vi "HEWH Flow Adjust Draw States.vi"(4 "GPM Target":T3=3.0 format="%.2f", 5 "Loop Rate":dbl, 6 "Elapsed Time (Sec)":dbl, 7 "Flow Selector":T1, 8 "Error In":errorcluster, 9 "Gallon Target":T3 format="%.2f", 10 "Core HEWH Data in":T4={"Scan Rate Adjust"=0.0, "Draw Count"=0, "Test Patten Setup"={"Total Gallons Schedule"=[], "PRAT/RLT Sequence"=[{"Sequence #"=1.0, "Cycles"=35, "Mode Setting"="", "Flow Rate (GPM)"=0.0, "Temperature (F)"=0.0, "Reset Timer"=FALSE, "Use Temp Decline Method"=FALSE, "Terminate Condition"=enum."C1-Terminate Draw @ Gallon Mark", "Condition Value #1"=0.0, "UE"=FALSE, "LE"=FALSE, "Comp"=FALSE, "Fan"=FALSE, "Test End Time (Sec)"=0.0, "Purge Until Cutout"=FALSE, "Start Conditions"=enum."Heat Source Cutout", "Condition Value #2"=0.0, "Remove Power"=FALSE, "Time"=0.0, "Check Special Cond."=enum."SC1-Do Nothing", "Condition#"=enum."C1", "Draw Flags"=enum."N/A", "Data Processing Delay (FHD 15sec, UEF 5 Sec)"=0.0, "Test Complete"=FALSE, "User Setpoint"=0.0, "Tank Setpoint"=0.0}, {"Sequence #"=2.0, "Cycles"=15, "Mode Setting"="", "Flow Rate (GPM)"=0.0, "Temperature (F)"=0.0, "Reset Timer"=FALSE, "Use Temp Decline Method"=FALSE, "Terminate Condition"=enum."C1-Terminate Draw @ Gallon Mark", "Condition Value #1"=0.0, "UE"=FALSE, "LE"=FALSE, "Comp"=FALSE, "Fan"=FALSE, "Test End Time (Sec)"=0.0, "Purge Until Cutout"=FALSE, "Start Conditions"=enum."Heat Source Cutout", "Condition Value #2"=0.0, "Remove Power"=FALSE, "Time"=0.0, "Check Special Cond."=enum."SC1-Do Nothing", "Condition#"=enum."C1", "Draw Flags"=enum."N/A", "Data Processing Delay (FHD 15sec, UEF 5 Sec)"=0.0, "Test Complete"=FALSE, "User Setpoint"=0.0, "Tank Setpoint"=0.0}, {"Sequence #"=3.0, "Cycles"=35, "Mode Setting"="", "Flow Rate (GPM)"=0.0, "Temperature (F)"=0.0, "Reset Timer"=FALSE, "Use Temp Decline Method"=FALSE, "Terminate Condition"=enum."C1-Terminate Draw @ Gallon Mark", "Condition Value #1"=0.0, "UE"=FALSE, "LE"=FALSE, "Comp"=FALSE, "Fan"=FALSE, "Test End Time (Sec)"=0.0, "Purge Until Cutout"=FALSE, "Start Conditions"=enum."Heat Source Cutout", "Condition Value #2"=0.0, "Remove Power"=FALSE, "Time"=0.0, "Check Special Cond."=enum."SC1-Do Nothing", "Condition#"=enum."C1", "Draw Flags"=enum."N/A", "Data Processing Delay (FHD 15sec, UEF 5 Sec)"=0.0, "Test Complete"=FALSE, "User Setpoint"=0.0, "Tank Setpoint"=0.0}, {"Sequence #"=4.0, "Cycles"=15, "Mode Setting"="", "Flow Rate (GPM)"=0.0, "Temperature (F)"=0.0, "Reset Timer"=FALSE, "Use Temp Decline Method"=FALSE, "Terminate Condition"=enum."C1-Terminate Draw @ Gallon Mark", "Condition Value #1"=0.0, "UE"=FALSE, "LE"=FALSE, "Comp"=FALSE, "Fan"=FALSE, "Test End Time (Sec)"=0.0, "Purge Until Cutout"=FALSE, "Start Conditions"=enum."Heat Source Cutout", "Condition Value #2"=0.0, "Remove Power"=FALSE, "Time"=0.0, "Check Special Cond."=enum."SC1-Do Nothing", "Condition#"=enum."C1", "Draw Flags"=enum."N/A", "Data Processing Delay (FHD 15sec, UEF 5 Sec)"=0.0, "Test Complete"=FALSE, "User Setpoint"=0.0, "Tank Setpoint"=0.0}, {"Sequence #"=5.0, "Cycles"=35, "Mode Setting"="", "Flow Rate (GPM)"=0.0, "Temperature (F)"=0.0, "Reset Timer"=FALSE, "Use Temp Decline Method"=FALSE, "Terminate Condition"=enum."C1-Terminate Draw @ Gallon Mark", "Condition Value #1"=0.0, "UE"=FALSE, "LE"=FALSE, "Comp"=FALSE, "Fan"=FALSE, "Test End Time (Sec)"=0.0, "Purge Until Cutout"=FALSE, "Start Conditions"=enum."Heat Source Cutout", "Condition Value #2"=0.0, "Remove Power"=FALSE, "Time"=0.0, "Check Special Cond."=enum."SC1-Do Nothing", "Condition#"=enum."C1", "Draw Flags"=enum."N/A", "Data Processing Delay (FHD 15sec, UEF 5 Sec)"=0.0, "Test Complete"=FALSE, "User Setpoint"=0.0, "Tank Setpoint"=0.0}, {"Sequence #"=6.0, "Cycles"=15, "Mode Setting"="", "Flow Rate (GPM)"=0.0, "Temperature (F)"=0.0, "Reset Timer"=FALSE, "Use Temp Decline Method"=FALSE, "Terminate Condition"=enum."C1-Terminate Draw @ Gallon Mark", "Condition Value #1"=0.0, "UE"=FALSE, "LE"=FALSE, "Comp"=FALSE, "Fan"=FALSE, "Test End Time (Sec)"=0.0, "Purge Until Cutout"=FALSE, "Start Conditions"=enum."Heat Source Cutout", "Condition Value #2"=0.0, "Remove Power"=FALSE, "Time"=0.0, "Check Special Cond."=enum."SC1-Do Nothing", "Condition#"=enum."C1", "Draw Flags"=enum."N/A", "Data Processing Delay (FHD 15sec, UEF 5 Sec)"=0.0, "Test Complete"=FALSE, "User Setpoint"=0.0, "Tank Setpoint"=0.0}, {"Sequence #"=7.0, "Cycles"=35, "Mode Setting"="", "Flow Rate (GPM)"=0.0, "Temperature (F)"=0.0, "Reset Timer"=FALSE, "Use Temp Decline Method"=FALSE, "Terminate Condition"=enum."C1-Terminate Draw @ Gallon Mark", "Condition Value #1"=0.0, "UE"=FALSE, "LE"=FALSE, "Comp"=FALSE, "Fan"=FALSE, "Test End Time (Sec)"=0.0, "Purge Until Cutout"=FALSE, "Start Conditions"=enum."Heat Source Cutout", "Condition Value #2"=0.0, "Remove Power"=FALSE, "Time"=0.0, "Check Special Cond."=enum."SC1-Do Nothing", "Condition#"=enum."C1", "Draw Flags"=enum."N/A", "Data Processing Delay (FHD 15sec, UEF 5 Sec)"=0.0, "Test Complete"=FALSE, "User Setpoint"=0.0, "Tank Setpoint"=0.0}, {"Sequence #"=8.0, "Cycles"=15, "Mode Setting"="", "Flow Rate (GPM)"=0.0, "Temperature (F)"=0.0, "Reset Timer"=FALSE, "Use Temp Decline Method"=FALSE, "Terminate Condition"=enum."C1-Terminate Draw @ Gallon Mark", "Condition Value #1"=0.0, "UE"=FALSE, "LE"=FALSE, "Comp"=FALSE, "Fan"=FALSE, "Test End Time (Sec)"=0.0, "Purge Until Cutout"=FALSE, "Start Conditions"=enum."Heat Source Cutout", "Condition Value #2"=0.0, "Remove Power"=FALSE, "Time"=0.0, "Check Special Cond."=enum."SC1-Do Nothing", "Condition#"=enum."C1", "Draw Flags"=enum."N/A", "Data Processing Delay (FHD 15sec, UEF 5 Sec)"=0.0, "Test Complete"=FALSE, "User Setpoint"=0.0, "Tank Setpoint"=0.0}], "Current Sequence Index"=0}, "HEWH Specific DAQ"={"HEWH Data"={"HEWH Standard"={"Voltage (Volts)"=0.0, "Current (Amps)"=0.0, "Power (Watts)"=0.0, "WattHours (Wh)"=0.0, "TC Tree (AVG)"=0.0, "Flow Rate (GPM)"=0.0, "Gallons (Gal)"=0.0, "RTD Out (Deg F)"=0.0, "RTD In (Deg F)"=0.0, "RTD Amb (Deg F)"=0.0, "TC Down"=0.0, "UE Event Lead"=0, "LE Event Lead"=0, "TC Tree Array"=[]}, "PRAT"={"Power (Watts) A"=4192.0, "Power (Watts) B"=4192.0, "Power (Watts) C"=4192.0, "Power (Watts) D"=4192.0, "TC1"=0.0, "TC2"=0.0, "TC3"=0.0, "TC4"=0.0, "WattHours (Wh) A"=4192.0, "WattHours (Wh) B"=4192.0, "WattHours (Wh) C"=4192.0, "WattHours (Wh) D"=4192.0, "Ambient"=0.0, "Extra Temp"=0.0}, "Additional Power Data"={"Vthd"=236.2, "Frequency (Hz)"=236.2, "Apparent Power (VA)"=236.2, "Power Factor"=236.2, "Current Crest Factor"=236.2, "Voltage Crest Factor"=236.2, "Integration Time (sec)"=236.2}}, "Flow Valve % Open"=0.0, "Power State"={"UE"=FALSE, "LE"=FALSE, "COMP"=FALSE, "FANS"=FALSE}, "Power Analyzer"=enum."", "Flow Valve uA Output"=0, "Gallons Start (Gal)"=0.0}, "Test Output Data"={"PreDraw Data Table"=[], "Data Table"=[], "MW100 TC Headers"=[]}, "Calc and Calibration"={"Mean SD Var Max Min Array"=[], "Draw Statistics (DBL)"=[], "Calibration Coefficients DBL"=[], "Start Gallons"=0.0, "Starting Temp Decline"=0.0, "K-Factor (Temperature)"=0.0, "All Draw Stats"=[], "RTD Terminate Value"=0.0, "K-Factor (Flow)"=0.0, "Intellifaucet Type"="", "Thermal Stabil Array"=[], "Gas Thermal Stabil Complete"=FALSE, "Therm Reset Cmpt 1"=FALSE, "Therm Reset Cmpt 2"=FALSE, "Last Flow Rate (Therm)"=0.0, "State"=enum."State 1", "Gas Thermal Time"=0.0, "Target Rate (Thermal)"=0.0, "Thermal - Final"=[], "State5 Gal Water"=0.0, "State 5 Gal Gas"=0.0, "Intellif Open < 1"=0.0, "Intellif Open < 1.7"=0.0, "Intellif Open < 2.2"=0.0, "Intellif Open > 2.2"=0.0, "End of Draw\nComparison"=[]}, "Current Draw Time"=0.0, "LV Program"=enum."HEWH", "Station ID"=enum."A", "Current Cond"=enum."N/A", "Test Complete"=FALSE, "ANSI Rate"={"Array 1"=[], "Array 3"=[], "Array 2"=[], "Start ANSI"=FALSE, "ANSI Start Time"=0.0, "Restart ANSI"=FALSE, "15 Min ANSI Avg (BTU/hr)"=0.0, "20 Min ANSI Avg (BTU/hr)"=0.0, "25 Min ANSI Avg (BTU/hr)"=0.0, "Absolute Pressure"=0.0, "Gas Temperature"=0.0, "Volumetric Flow Rate"=0.0, "Mass Flow Rate"=0.0, "Array 4"=[], "Array 5"=[], "Gas Rate"=0.0, "15 Min Pres Avg (PSIA)"=0.0, "20 Min Pres Avg (PSIA)"=0.0, "25 Min Pres Avg (PSIA)"=0.0, "15 Min Temp Avg (°F) "=0.0, "20 Min Temp Avg (°F)"=0.0, "25 Min Temp Avg (°F)"=0.0, "15 Min Uncorrected Avg (CFH)"=0.0, "20 Min Uncorrected Avg (CFH)"=0.0, "25 Min Uncorrected Avg (CFH)"=0.0, "15 Min Corrected Avg (SCFH)"=0.0, "20 Min Corrected Avg (SCFH)"=0.0, "25 Min Corrected Avg (SCFH)"=0.0, "15 Min Complete"=FALSE, "20 Min Complete"=FALSE, "25 Min Complete"=FALSE, "Heating Value (BTU/ft³)"=0.0, "CO CO2 15 Min"=[], "CO CO2 20 Min"=[], "CO CO2 25 Min"=[], "CO CO2 Real Time"=[]}, "Gas Measurment Data"={"Absolute Pressure"=0.0, "Gauge/Diff. Pressure"=0.0, "Barometric Pressure"=0.0, "Temperature"=0.0, "Volumetric Flow"=0.0, "Mass Flow"=0.0, "Setpoint"=0.0, "Valve Drive"=0.0, "Totalizer"=0.0, "[hr]"=0.0, "[min]"=0.0, "[sec]"=0.0, "Totalizer Average Flow"=0.0, "Totalizer Peak Flow"=0.0, "Gas selected"=""}, "Module 4 Relay Status"={"INTELLIFAUCET TEMP(T)/FLOW(F) (CH 041)"=FALSE, "INTELLIFAUCET READY (CH 042)"=FALSE, "INTELLIFAUCET START (CH 043)"=FALSE, "INTELLIFAUCET STOP (CH 044)"=FALSE, "MAIN POWER RELAY (CH 047)"=FALSE, "NOT USED (CH 045)"=FALSE, "NOT USED (CH 046)"=FALSE, "PURGE VALVE RELAY (CH 048)"=FALSE, "OUTLET VALVE RELAY (CH 049)"=FALSE, "INLET VALVE RELAY (CH 050)"=FALSE, "Intellifaucet (% Open)"=0.0, "Proportioning Valve (%Open)"=0.0, "Intellifaucet Temp Setpoint (F)"=0.0}, "Inficon Data Output"={"Gross Heating Value, Vol (Real, Dry)"=1067.4462890625, "Nitrogen Component Normalized Mole % (Dry)"=0.0, "Methane Component Normalized Mole % (Dry)"=92.87550354003906, "Carbon Dioxide Component Normalized Mole % (Dry)"=0.1941000074148178, "Ethane Component Normalized Mole % (Dry)"=6.454999923706055, "Propane Component Normalized Mole % (Dry)"=0.3865000009536743, "i-Pentane Component Normalized Mole % (Dry)"=0.007799999788403511, "i-Butane Component Normalized Mole % (Dry)"=0.03880000114440918, "n-Butane Component Normalized Mole % (Dry)"=0.03819999843835831, "n-Pentane Component Normalized Mole % (Dry)"=0.004100000020116568, "Hexane Component Normalized Mole % (Dry)"=0.0, "Heptane Component Normalized Mole % (Dry)"=0.0, "Gross Wobbe Index, Real(Dry)"=1385.8905029296875, "Relative Density, Real(Dry)"=0.5932452082633972, "Propylene Component Normalized Mole % (Dry)"=0.0, "C4 Olefins Component Normalized Mole % (Dry)"=0.0, "Water Component Normalized Mole % (Dry)"=0.0}} {"Test Patten Setup"."PRAT/RLT Sequence"."Time" format="%<%H:%M:%S>t"; "Test Patten Setup"."Total Gallons Schedule" format="%.2f"}, 11 "Emerson Flow Meter Data Input":T2) -> (0 "Error Out":errorcluster, 1 "Time to Draw Water (Seconds)":T3 format="%.2f", 2 "Core HEWH Data (Out)":T4={"Scan Rate Adjust"=0.0, "Draw Count"=0, "Test Patten Setup"={"Total Gallons Schedule"=[], "PRAT/RLT Sequence"=[{"Sequence #"=1.0, "Cycles"=35, "Mode Setting"="", "Flow Rate (GPM)"=0.0, "Temperature (F)"=0.0, "Reset Timer"=FALSE, "Use Temp Decline Method"=FALSE, "Terminate Condition"=enum."C1-Terminate Draw @ Gallon Mark", "Condition Value #1"=0.0, "UE"=FALSE, "LE"=FALSE, "Comp"=FALSE, "Fan"=FALSE, "Test End Time (Sec)"=0.0, "Purge Until Cutout"=FALSE, "Start Conditions"=enum."Heat Source Cutout", "Condition Value #2"=0.0, "Remove Power"=FALSE, "Time"=0.0, "Check Special Cond."=enum."SC1-Do Nothing", "Condition#"=enum."C1", "Draw Flags"=enum."N/A", "Data Processing Delay (FHD 15sec, UEF 5 Sec)"=0.0, "Test Complete"=FALSE, "User Setpoint"=0.0, "Tank Setpoint"=0.0}, {"Sequence #"=2.0, "Cycles"=15, "Mode Setting"="", "Flow Rate (GPM)"=0.0, "Temperature (F)"=0.0, "Reset Timer"=FALSE, "Use Temp Decline Method"=FALSE, "Terminate Condition"=enum."C1-Terminate Draw @ Gallon Mark", "Condition Value #1"=0.0, "UE"=FALSE, "LE"=FALSE, "Comp"=FALSE, "Fan"=FALSE, "Test End Time (Sec)"=0.0, "Purge Until Cutout"=FALSE, "Start Conditions"=enum."Heat Source Cutout", "Condition Value #2"=0.0, "Remove Power"=FALSE, "Time"=0.0, "Check Special Cond."=enum."SC1-Do Nothing", "Condition#"=enum."C1", "Draw Flags"=enum."N/A", "Data Processing Delay (FHD 15sec, UEF 5 Sec)"=0.0, "Test Complete"=FALSE, "User Setpoint"=0.0, "Tank Setpoint"=0.0}, {"Sequence #"=3.0, "Cycles"=35, "Mode Setting"="", "Flow Rate (GPM)"=0.0, "Temperature (F)"=0.0, "Reset Timer"=FALSE, "Use Temp Decline Method"=FALSE, "Terminate Condition"=enum."C1-Terminate Draw @ Gallon Mark", "Condition Value #1"=0.0, "UE"=FALSE, "LE"=FALSE, "Comp"=FALSE, "Fan"=FALSE, "Test End Time (Sec)"=0.0, "Purge Until Cutout"=FALSE, "Start Conditions"=enum."Heat Source Cutout", "Condition Value #2"=0.0, "Remove Power"=FALSE, "Time"=0.0, "Check Special Cond."=enum."SC1-Do Nothing", "Condition#"=enum."C1", "Draw Flags"=enum."N/A", "Data Processing Delay (FHD 15sec, UEF 5 Sec)"=0.0, "Test Complete"=FALSE, "User Setpoint"=0.0, "Tank Setpoint"=0.0}, {"Sequence #"=4.0, "Cycles"=15, "Mode Setting"="", "Flow Rate (GPM)"=0.0, "Temperature (F)"=0.0, "Reset Timer"=FALSE, "Use Temp Decline Method"=FALSE, "Terminate Condition"=enum."C1-Terminate Draw @ Gallon Mark", "Condition Value #1"=0.0, "UE"=FALSE, "LE"=FALSE, "Comp"=FALSE, "Fan"=FALSE, "Test End Time (Sec)"=0.0, "Purge Until Cutout"=FALSE, "Start Conditions"=enum."Heat Source Cutout", "Condition Value #2"=0.0, "Remove Power"=FALSE, "Time"=0.0, "Check Special Cond."=enum."SC1-Do Nothing", "Condition#"=enum."C1", "Draw Flags"=enum."N/A", "Data Processing Delay (FHD 15sec, UEF 5 Sec)"=0.0, "Test Complete"=FALSE, "User Setpoint"=0.0, "Tank Setpoint"=0.0}, {"Sequence #"=5.0, "Cycles"=35, "Mode Setting"="", "Flow Rate (GPM)"=0.0, "Temperature (F)"=0.0, "Reset Timer"=FALSE, "Use Temp Decline Method"=FALSE, "Terminate Condition"=enum."C1-Terminate Draw @ Gallon Mark", "Condition Value #1"=0.0, "UE"=FALSE, "LE"=FALSE, "Comp"=FALSE, "Fan"=FALSE, "Test End Time (Sec)"=0.0, "Purge Until Cutout"=FALSE, "Start Conditions"=enum."Heat Source Cutout", "Condition Value #2"=0.0, "Remove Power"=FALSE, "Time"=0.0, "Check Special Cond."=enum."SC1-Do Nothing", "Condition#"=enum."C1", "Draw Flags"=enum."N/A", "Data Processing Delay (FHD 15sec, UEF 5 Sec)"=0.0, "Test Complete"=FALSE, "User Setpoint"=0.0, "Tank Setpoint"=0.0}, {"Sequence #"=6.0, "Cycles"=15, "Mode Setting"="", "Flow Rate (GPM)"=0.0, "Temperature (F)"=0.0, "Reset Timer"=FALSE, "Use Temp Decline Method"=FALSE, "Terminate Condition"=enum."C1-Terminate Draw @ Gallon Mark", "Condition Value #1"=0.0, "UE"=FALSE, "LE"=FALSE, "Comp"=FALSE, "Fan"=FALSE, "Test End Time (Sec)"=0.0, "Purge Until Cutout"=FALSE, "Start Conditions"=enum."Heat Source Cutout", "Condition Value #2"=0.0, "Remove Power"=FALSE, "Time"=0.0, "Check Special Cond."=enum."SC1-Do Nothing", "Condition#"=enum."C1", "Draw Flags"=enum."N/A", "Data Processing Delay (FHD 15sec, UEF 5 Sec)"=0.0, "Test Complete"=FALSE, "User Setpoint"=0.0, "Tank Setpoint"=0.0}, {"Sequence #"=7.0, "Cycles"=35, "Mode Setting"="", "Flow Rate (GPM)"=0.0, "Temperature (F)"=0.0, "Reset Timer"=FALSE, "Use Temp Decline Method"=FALSE, "Terminate Condition"=enum."C1-Terminate Draw @ Gallon Mark", "Condition Value #1"=0.0, "UE"=FALSE, "LE"=FALSE, "Comp"=FALSE, "Fan"=FALSE, "Test End Time (Sec)"=0.0, "Purge Until Cutout"=FALSE, "Start Conditions"=enum."Heat Source Cutout", "Condition Value #2"=0.0, "Remove Power"=FALSE, "Time"=0.0, "Check Special Cond."=enum."SC1-Do Nothing", "Condition#"=enum."C1", "Draw Flags"=enum."N/A", "Data Processing Delay (FHD 15sec, UEF 5 Sec)"=0.0, "Test Complete"=FALSE, "User Setpoint"=0.0, "Tank Setpoint"=0.0}, {"Sequence #"=8.0, "Cycles"=15, "Mode Setting"="", "Flow Rate (GPM)"=0.0, "Temperature (F)"=0.0, "Reset Timer"=FALSE, "Use Temp Decline Method"=FALSE, "Terminate Condition"=enum."C1-Terminate Draw @ Gallon Mark", "Condition Value #1"=0.0, "UE"=FALSE, "LE"=FALSE, "Comp"=FALSE, "Fan"=FALSE, "Test End Time (Sec)"=0.0, "Purge Until Cutout"=FALSE, "Start Conditions"=enum."Heat Source Cutout", "Condition Value #2"=0.0, "Remove Power"=FALSE, "Time"=0.0, "Check Special Cond."=enum."SC1-Do Nothing", "Condition#"=enum."C1", "Draw Flags"=enum."N/A", "Data Processing Delay (FHD 15sec, UEF 5 Sec)"=0.0, "Test Complete"=FALSE, "User Setpoint"=0.0, "Tank Setpoint"=0.0}], "Current Sequence Index"=0}, "HEWH Specific DAQ"={"HEWH Data"={"HEWH Standard"={"Voltage (Volts)"=0.0, "Current (Amps)"=0.0, "Power (Watts)"=0.0, "WattHours (Wh)"=0.0, "TC Tree (AVG)"=0.0, "Flow Rate (GPM)"=0.0, "Gallons (Gal)"=0.0, "RTD Out (Deg F)"=0.0, "RTD In (Deg F)"=0.0, "RTD Amb (Deg F)"=0.0, "TC Down"=0.0, "UE Event Lead"=0, "LE Event Lead"=0, "TC Tree Array"=[]}, "PRAT"={"Power (Watts) A"=4192.0, "Power (Watts) B"=4192.0, "Power (Watts) C"=4192.0, "Power (Watts) D"=4192.0, "TC1"=0.0, "TC2"=0.0, "TC3"=0.0, "TC4"=0.0, "WattHours (Wh) A"=4192.0, "WattHours (Wh) B"=4192.0, "WattHours (Wh) C"=4192.0, "WattHours (Wh) D"=4192.0, "Ambient"=0.0, "Extra Temp"=0.0}, "Additional Power Data"={"Vthd"=236.2, "Frequency (Hz)"=236.2, "Apparent Power (VA)"=236.2, "Power Factor"=236.2, "Current Crest Factor"=236.2, "Voltage Crest Factor"=236.2, "Integration Time (sec)"=236.2}}, "Flow Valve % Open"=0.0, "Power State"={"UE"=FALSE, "LE"=FALSE, "COMP"=FALSE, "FANS"=FALSE}, "Power Analyzer"=enum."", "Flow Valve uA Output"=0, "Gallons Start (Gal)"=0.0}, "Test Output Data"={"PreDraw Data Table"=[], "Data Table"=[], "MW100 TC Headers"=[]}, "Calc and Calibration"={"Mean SD Var Max Min Array"=[], "Draw Statistics (DBL)"=[], "Calibration Coefficients DBL"=[], "Start Gallons"=0.0, "Starting Temp Decline"=0.0, "K-Factor (Temperature)"=0.0, "All Draw Stats"=[], "RTD Terminate Value"=0.0, "K-Factor (Flow)"=0.0, "Intellifaucet Type"="", "Thermal Stabil Array"=[], "Gas Thermal Stabil Complete"=FALSE, "Therm Reset Cmpt 1"=FALSE, "Therm Reset Cmpt 2"=FALSE, "Last Flow Rate (Therm)"=0.0, "State"=enum."State 1", "Gas Thermal Time"=0.0, "Target Rate (Thermal)"=0.0, "Thermal - Final"=[], "State5 Gal Water"=0.0, "State 5 Gal Gas"=0.0, "Intellif Open < 1"=0.0, "Intellif Open < 1.7"=0.0, "Intellif Open < 2.2"=0.0, "Intellif Open > 2.2"=0.0, "End of Draw\nComparison"=[]}, "Current Draw Time"=0.0, "LV Program"=enum."HEWH", "Station ID"=enum."A", "Current Cond"=enum."N/A", "Test Complete"=FALSE, "ANSI Rate"={"Array 1"=[], "Array 3"=[], "Array 2"=[], "Start ANSI"=FALSE, "ANSI Start Time"=0.0, "Restart ANSI"=FALSE, "15 Min ANSI Avg (BTU/hr)"=0.0, "20 Min ANSI Avg (BTU/hr)"=0.0, "25 Min ANSI Avg (BTU/hr)"=0.0, "Absolute Pressure"=0.0, "Gas Temperature"=0.0, "Volumetric Flow Rate"=0.0, "Mass Flow Rate"=0.0, "Array 4"=[], "Array 5"=[], "Gas Rate"=0.0, "15 Min Pres Avg (PSIA)"=0.0, "20 Min Pres Avg (PSIA)"=0.0, "25 Min Pres Avg (PSIA)"=0.0, "15 Min Temp Avg (°F) "=0.0, "20 Min Temp Avg (°F)"=0.0, "25 Min Temp Avg (°F)"=0.0, "15 Min Uncorrected Avg (CFH)"=0.0, "20 Min Uncorrected Avg (CFH)"=0.0, "25 Min Uncorrected Avg (CFH)"=0.0, "15 Min Corrected Avg (SCFH)"=0.0, "20 Min Corrected Avg (SCFH)"=0.0, "25 Min Corrected Avg (SCFH)"=0.0, "15 Min Complete"=FALSE, "20 Min Complete"=FALSE, "25 Min Complete"=FALSE, "Heating Value (BTU/ft³)"=0.0, "CO CO2 15 Min"=[], "CO CO2 20 Min"=[], "CO CO2 25 Min"=[], "CO CO2 Real Time"=[]}, "Gas Measurment Data"={"Absolute Pressure"=0.0, "Gauge/Diff. Pressure"=0.0, "Barometric Pressure"=0.0, "Temperature"=0.0, "Volumetric Flow"=0.0, "Mass Flow"=0.0, "Setpoint"=0.0, "Valve Drive"=0.0, "Totalizer"=0.0, "[hr]"=0.0, "[min]"=0.0, "[sec]"=0.0, "Totalizer Average Flow"=0.0, "Totalizer Peak Flow"=0.0, "Gas selected"=""}, "Module 4 Relay Status"={"INTELLIFAUCET TEMP(T)/FLOW(F) (CH 041)"=FALSE, "INTELLIFAUCET READY (CH 042)"=FALSE, "INTELLIFAUCET START (CH 043)"=FALSE, "INTELLIFAUCET STOP (CH 044)"=FALSE, "MAIN POWER RELAY (CH 047)"=FALSE, "NOT USED (CH 045)"=FALSE, "NOT USED (CH 046)"=FALSE, "PURGE VALVE RELAY (CH 048)"=FALSE, "OUTLET VALVE RELAY (CH 049)"=FALSE, "INLET VALVE RELAY (CH 050)"=FALSE, "Intellifaucet (% Open)"=0.0, "Proportioning Valve (%Open)"=0.0, "Intellifaucet Temp Setpoint (F)"=0.0}, "Inficon Data Output"={"Gross Heating Value, Vol (Real, Dry)"=1067.4462890625, "Nitrogen Component Normalized Mole % (Dry)"=0.0, "Methane Component Normalized Mole % (Dry)"=92.87550354003906, "Carbon Dioxide Component Normalized Mole % (Dry)"=0.1941000074148178, "Ethane Component Normalized Mole % (Dry)"=6.454999923706055, "Propane Component Normalized Mole % (Dry)"=0.3865000009536743, "i-Pentane Component Normalized Mole % (Dry)"=0.007799999788403511, "i-Butane Component Normalized Mole % (Dry)"=0.03880000114440918, "n-Butane Component Normalized Mole % (Dry)"=0.03819999843835831, "n-Pentane Component Normalized Mole % (Dry)"=0.004100000020116568, "Hexane Component Normalized Mole % (Dry)"=0.0, "Heptane Component Normalized Mole % (Dry)"=0.0, "Gross Wobbe Index, Real(Dry)"=1385.8905029296875, "Relative Density, Real(Dry)"=0.5932452082633972, "Propylene Component Normalized Mole % (Dry)"=0.0, "C4 Olefins Component Normalized Mole % (Dry)"=0.0, "Water Component Normalized Mole % (Dry)"=0.0}} {"Test Patten Setup"."PRAT/RLT Sequence"."Time" format="%<%H:%M:%S>t"; "Test Patten Setup"."Total Gallons Schedule" format="%.2f"}, 3 "Terminate":bool)   [LabVIEW 2019]
uses:
  Type Definitions/HEWH Output Information.ctl
  Type Definitions/HEWH Draw Pattern Setup.ctl
  Type Definitions/PRAT Test.ctl
  Utility/Save File/File Setup (Public)/Type Definition/Save File HEWH Heating Control Mode.ctl
  Type Definitions/Terminate Draw Conditions.ctl
  Type Definitions/HEWH Start Conditions.ctl
  Type Definitions/Check Special Condtions.ctl
  Type Definitions/HEWH Special Condition Check.ctl
  Type Definitions/HEWH Draw Flag ENUM.ctl
  Type Definitions/HEWH Specific DAQ.ctl
  Type Definitions/HEWH Power Data.ctl
  Type Definitions/HEWH Power Elements.ctl
  Utility/Type Definitions/UTILITY Power Analyzer.ctl
  Type Definitions/HEWH Calc and Calibration.ctl
  Utility/Save File/File Setup (Public)/Type Definition/Save File DOE LabView Program.ctl
  Custom Instrument Control/MW100/Type Definitions/Station ID Selector.ctl
  Range/Type Definitions/RANGE ANSI Rate.ctl
  Drivers/Alicat Gas Meter Driver/Sub-VIs/Data Cluster.ctl
  Custom Instrument Control/MW100/Type Definitions/HEWH Module 4 Relay Status.ctl
  Drivers/Inficon Fusion Micro GC/Type Definitions/Inficon Data.ctl
  Utility/Custom Pallet Controls/Custom Pallet DBL.ctl
  Drivers/Emerson 5700 Transmitter/Type Definitions/Emerson 5700 Data.ctl
  Type Definitions/Flow Meter Selector.ctl
  Utility/Type Definitions/UTILITY Notifier.ctl
  Utility/Save File/File Setup.lvlib
panel:
  # "Natural Gas"
  # "Propane"
  # "Totalizer Timer"
  # "Draw Pattern Setup (24 Hour)"
  # "Natural Gas"
  # "Propane"
  # "Totalizer Timer"
  # "Draw Pattern Setup (24 Hour)"
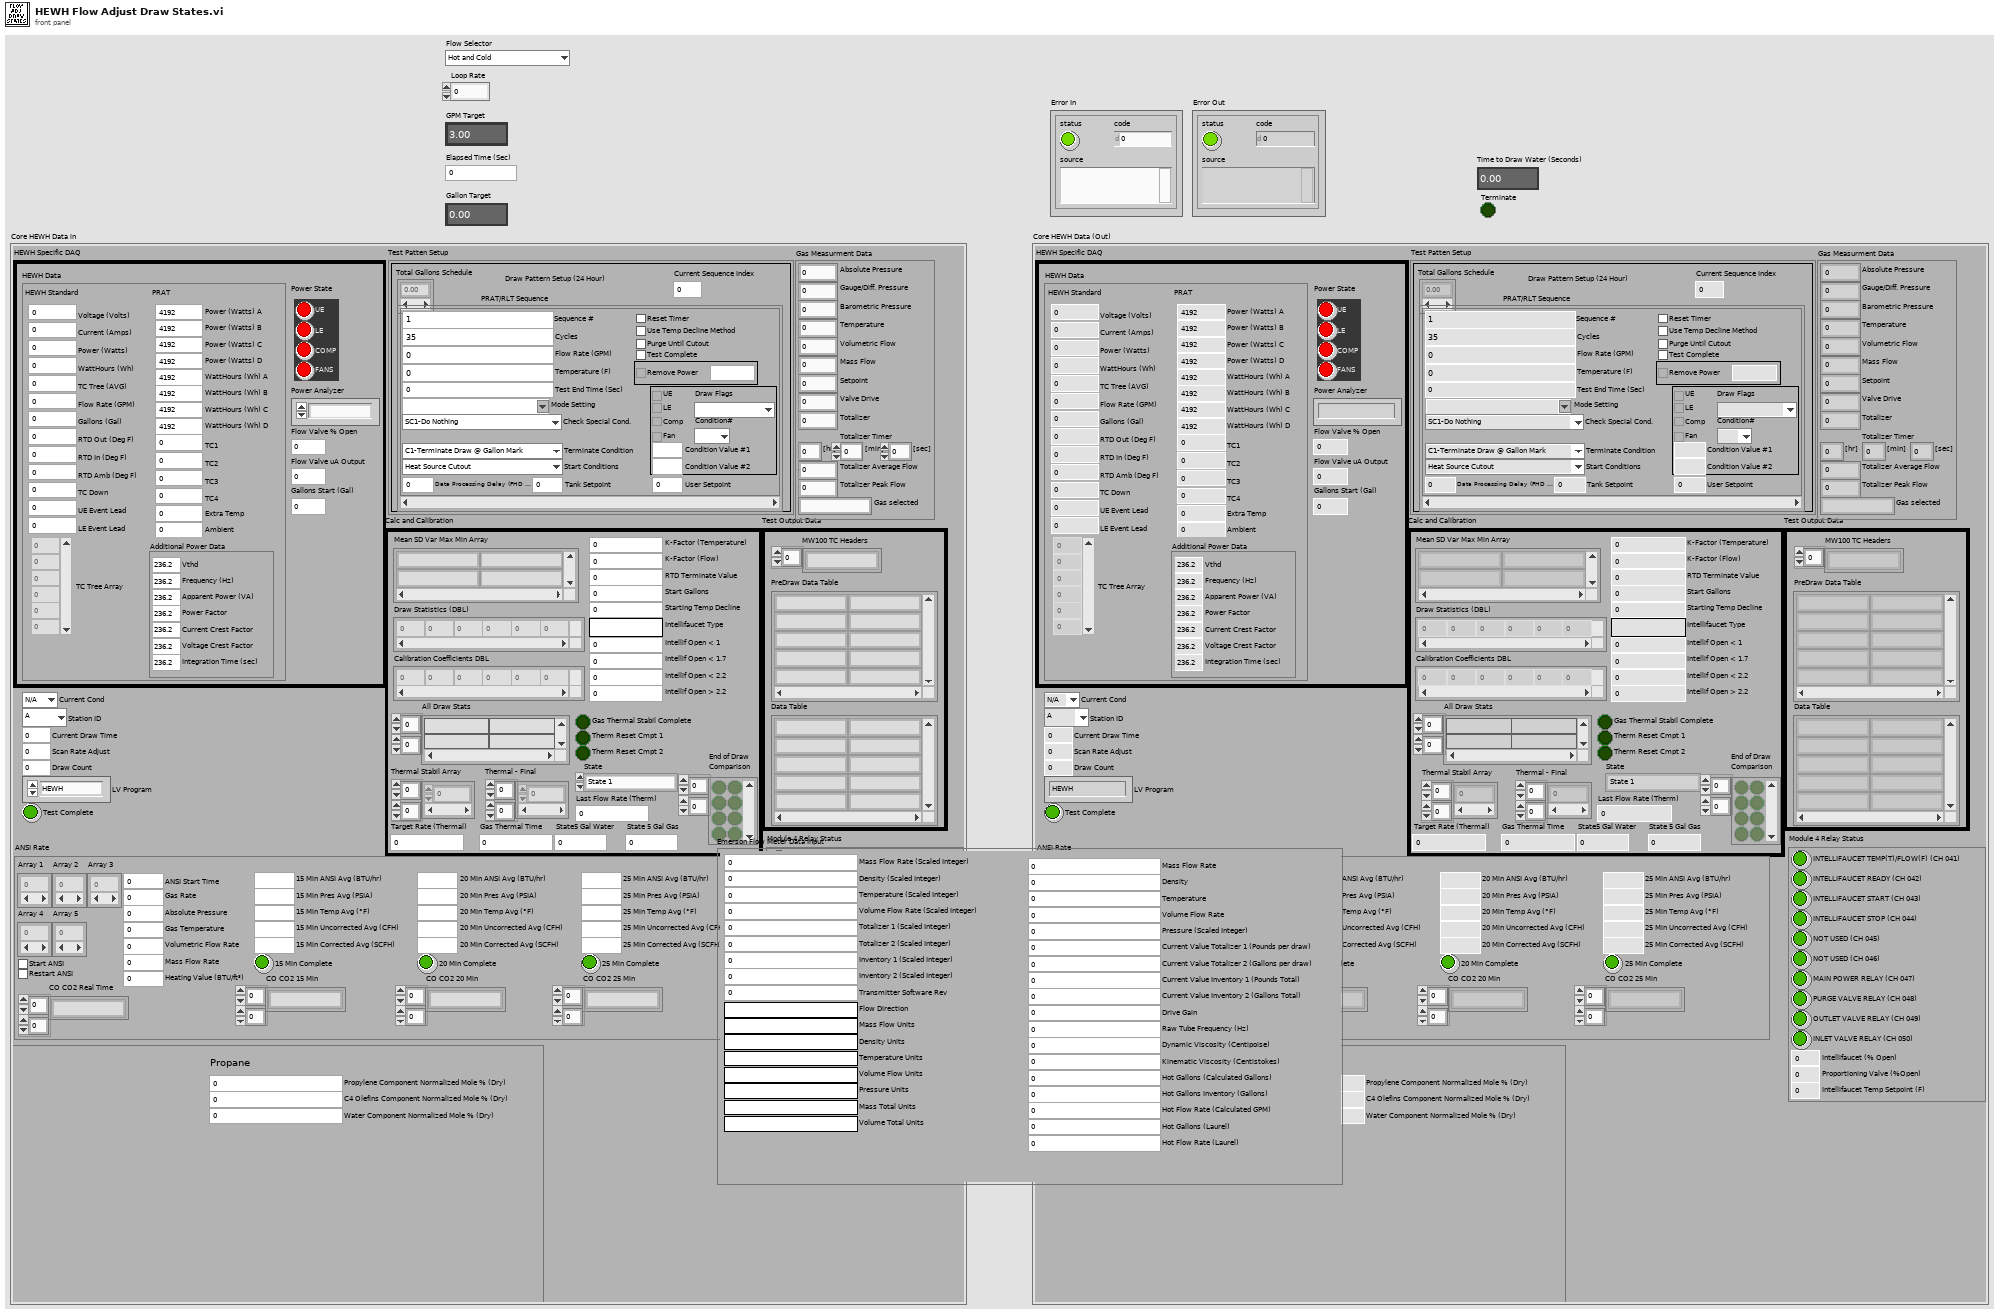
[diagram p1: front panel]
types:
  T1 = typedef "Flow Meter Selector.ctl" = enum16{"Hot and Cold", "Hot", "Cold", "None"}
  T2 = typedef "Emerson 5700 Data.ctl" = cluster{"Mass Flow Rate (Scaled Integer)":u16, "Density (Scaled Integer)":u16, "Temperature (Scaled Integer)":u16, "Volume Flow Rate (Scaled Integer)":u16, "Totalizer 1 (Scaled Integer)":u16, "Totalizer 2 (Scaled Integer)":u16, "Transmitter Software Rev":u16, "Flow Direction":string, "Mass Flow Units":string, "Density Units":string, "Temperature Units":string, "Volume Flow Units":string, "Pressure Units":string, "Mass Total Units":string, "Volume Total Units":string, "Inventory 1 (Scaled Integer)":u16, "Inventory 2 (Scaled Integer)":u16, "Mass Flow Rate":dbl, "Density":dbl, "Temperature":dbl, "Volume Flow Rate":dbl, "Pressure (Scaled Integer)":u16, "Current Value Totalizer 1 (Pounds per draw)":dbl, "Current Value Totalizer 2 (Gallons per draw)":dbl, "Current Value Inventory 1 (Pounds Total)":dbl, "Current Value Inventory 2 (Gallons Total)":dbl, "Drive Gain":dbl, "Raw Tube Frequency (Hz)":dbl, "Dynamic Viscosity (Centipoise)":dbl, "Kinematic Viscosity (Centistokes)":dbl, "Hot Gallons (Calculated Gallons)":dbl, "Hot Flow Rate (Calculated GPM)":dbl, "Hot Gallons Inventory (Gallons)":dbl, "Hot Flow Rate (Laurel)":dbl, "Hot Gallons (Laurel)":dbl}
  T3 = typedef "Custom Pallet DBL.ctl" = dbl
  T4 = typedef "HEWH Output Information.ctl" = cluster{"Scan Rate Adjust":dbl, "Draw Count":i32, "Test Patten Setup":T5, "HEWH Specific DAQ":T13, "Test Output Data":cluster{"PreDraw Data Table":string[][], "Data Table":string[][], "MW100 TC Headers":string[]}, "Calc and Calibration":T17, "Current Draw Time":dbl, "LV Program":T18, "Station ID":T19, "Current Cond":T11, "Test Complete":bool, "ANSI Rate":T20, "Gas Measurment Data":T21, "Module 4 Relay Status":T22, "Inficon Data Output":T23}
  T5 = typedef "HEWH Draw Pattern Setup.ctl" = cluster{"Total Gallons Schedule":dbl[], "PRAT/RLT Sequence":T6[], "Current Sequence Index":i32}
  T6 = typedef "PRAT Test.ctl" = cluster{"Sequence #":dbl, "Cycles":i32, "Mode Setting":T7, "Flow Rate (GPM)":dbl, "Temperature (F)":dbl, "Reset Timer":bool, "Use Temp Decline Method":bool, "Terminate Condition":T8, "Condition Value #1":dbl, "UE":bool, "LE":bool, "Comp":bool, "Fan":bool, "Test End Time (Sec)":dbl, "Purge Until Cutout":bool, "Start Conditions":T9, "Condition Value #2":dbl, "Remove Power":bool, "Time":dbl, "Check Special Cond.":T10, "Condition#":T11, "Draw Flags":T12, "Data Processing Delay (FHD 15sec, UEF 5 Sec)":dbl, "Test Complete":bool, "User Setpoint":dbl, "Tank Setpoint":dbl}
  T7 = typedef "File Setup.lvlib/Save File HEWH Heating Control Mode.ctl" = string
  T8 = typedef "Terminate Draw Conditions.ctl" = enum16{"C1-Terminate Draw @ Gallon Mark", "C2-Special Last Draw (HU Test)", "C3-RTD Out <=", "C4-Mean Tank Temp <=", "C5-Decrease RTD Out (Deg F)", "C6-Time (Seconds)", "C7-Until Any Heat Source", "C8-Specific Heat Source", "C9-Do Nothing", "C10-Inlet Outlet RTD Temp Delta"}
  T9 = typedef "HEWH Start Conditions.ctl" = enum16{"Heat Source Cutout", "At Time (Seconds)", "Every X (Seconds)", "T2 >= X° Below Setpoint", "Seconds From Complete", "Wait for LE & Comp Cutout", "Wait for Comp Cutout", "Wait for LE Cutout", "Wait for UE Cutout", "Start Immediately"}
  T10 = typedef "Check Special Condtions.ctl" = enum16{"SC1-Do Nothing", "SC2-Check Heat Source (On-C2/Off-C1)", "SC3-Check Skip Condition", "SC4-Check Heat Source ON/Fail", "SC5-Keep Draw Valves Open", "SC6-Skip Purge"}
  T11 = typedef "HEWH Special Condition Check.ctl" = enum16{"N/A", "C1", "C2", "Reset/Fail", "Skip Draw Sequence"}
  T12 = typedef "HEWH Draw Flag ENUM.ctl" = enum16{"N/A", "None(0)", "Sml(1)", "Med(2)", "SmlMed(3)", "Lrg(4)", "SmlLrg(5)", "MedLrg(6)", "SmlMedLrg(7)"}
  T13 = typedef "HEWH Specific DAQ.ctl" = cluster{"HEWH Data":T14, "Flow Valve % Open":dbl, "Power State":T15, "Power Analyzer":T16, "Flow Valve uA Output":i32, "Gallons Start (Gal)":dbl}
  T14 = typedef "HEWH Power Data.ctl" = cluster{"HEWH Standard":cluster{"Voltage (Volts)":dbl, "Current (Amps)":dbl, "Power (Watts)":dbl, "WattHours (Wh)":dbl, "TC Tree (AVG)":dbl, "Flow Rate (GPM)":dbl, "Gallons (Gal)":dbl, "RTD Out (Deg F)":dbl, "RTD In (Deg F)":dbl, "RTD Amb (Deg F)":dbl, "TC Down":dbl, "UE Event Lead":i32, "LE Event Lead":i32, "TC Tree Array":dbl[]}, "PRAT":cluster{"Power (Watts) A":dbl, "Power (Watts) B":dbl, "Power (Watts) C":dbl, "Power (Watts) D":dbl, "TC1":dbl, "TC2":dbl, "TC3":dbl, "TC4":dbl, "WattHours (Wh) A":dbl, "WattHours (Wh) B":dbl, "WattHours (Wh) C":dbl, "WattHours (Wh) D":dbl, "Ambient":dbl, "Extra Temp":dbl}, "Additional Power Data":cluster{"Vthd":dbl, "Frequency (Hz)":dbl, "Apparent Power (VA)":dbl, "Power Factor":dbl, "Current Crest Factor":dbl, "Voltage Crest Factor":dbl, "Integration Time (sec)":dbl}}
  T15 = typedef "HEWH Power Elements.ctl" = cluster{"UE":bool, "LE":bool, "COMP":bool, "FANS":bool}
  T16 = typedef "UTILITY Power Analyzer.ctl" = enum16{"", "APLUS", "WT210", "WT500", "WT300", "OSI", "Debug", "WT230", "WT300_1", "WT300_2"}
  T17 = typedef "HEWH Calc and Calibration.ctl" = cluster{"Mean SD Var Max Min Array":string[][], "Draw Statistics (DBL)":dbl[][], "Calibration Coefficients DBL":dbl[][], "Start Gallons":dbl, "Starting Temp Decline":dbl, "K-Factor (Temperature)":dbl, "All Draw Stats":string[][], "RTD Terminate Value":dbl, "K-Factor (Flow)":dbl, "Intellifaucet Type":string, "Thermal Stabil Array":dbl[][], "Gas Thermal Stabil Complete":bool, "Therm Reset Cmpt 1":bool, "Therm Reset Cmpt 2":bool, "Last Flow Rate (Therm)":dbl, "State":enum16{"State 0", "State 1", "State 2", "State 3", "State 4", "State 5", "State 6"}, "Gas Thermal Time":dbl, "Target Rate (Thermal)":dbl, "Thermal - Final":dbl[][], "State5 Gal Water":dbl, "State 5 Gal Gas":dbl, "Intellif Open < 1":dbl, "Intellif Open < 1.7":dbl, "Intellif Open < 2.2":dbl, "Intellif Open > 2.2":dbl, "End of Draw\nComparison":bool[][]}
  T18 = typedef "File Setup.lvlib/Save File DOE LabView Program.ctl" = enum16{"No Name Found", "DOE Stand", "Dishwasher Kitchen", "Portable Stand", "HEWH", "Dryer", "Dryer WILT", "HCC", "PRAT", "HEWH RLT", "Refrigeration", "Gas Water Heater"}
  T19 = typedef "Station ID Selector.ctl" = enum16{"", "A", "B", "C", "D", "Global"}
  T20 = typedef "RANGE ANSI Rate.ctl" = cluster{"Array 1":dbl[], "Array 3":dbl[], "Array 2":dbl[], "Start ANSI":bool, "ANSI Start Time":dbl, "Restart ANSI":bool, "15 Min ANSI Avg (BTU/hr)":dbl, "20 Min ANSI Avg (BTU/hr)":dbl, "25 Min ANSI Avg (BTU/hr)":dbl, "Absolute Pressure":dbl, "Gas Temperature":dbl, "Volumetric Flow Rate":dbl, "Mass Flow Rate":dbl, "Array 4":dbl[], "Array 5":dbl[], "Gas Rate":dbl, "15 Min Pres Avg (PSIA)":dbl, "20 Min Pres Avg (PSIA)":dbl, "25 Min Pres Avg (PSIA)":dbl, "15 Min Temp Avg (°F) ":dbl, "20 Min Temp Avg (°F)":dbl, "25 Min Temp Avg (°F)":dbl, "15 Min Uncorrected Avg (CFH)":dbl, "20 Min Uncorrected Avg (CFH)":dbl, "25 Min Uncorrected Avg (CFH)":dbl, "15 Min Corrected Avg (SCFH)":dbl, "20 Min Corrected Avg (SCFH)":dbl, "25 Min Corrected Avg (SCFH)":dbl, "15 Min Complete":bool, "20 Min Complete":bool, "25 Min Complete":bool, "Heating Value (BTU/ft³)":dbl, "CO CO2 15 Min":string[][], "CO CO2 20 Min":string[][], "CO CO2 25 Min":string[][], "CO CO2 Real Time":string[][]}
  T21 = typedef "Data Cluster.ctl" = cluster{"Absolute Pressure":dbl, "Gauge/Diff. Pressure":dbl, "Barometric Pressure":dbl, "Temperature":dbl, "Volumetric Flow":dbl, "Mass Flow":dbl, "Setpoint":dbl, "Valve Drive":dbl, "Totalizer":dbl, "[hr]":dbl, "[min]":dbl, "[sec]":dbl, "Totalizer Average Flow":dbl, "Totalizer Peak Flow":dbl, "Gas selected":string}
  T22 = typedef "HEWH Module 4 Relay Status.ctl" = cluster{"INTELLIFAUCET TEMP(T)/FLOW(F) (CH 041)":bool, "INTELLIFAUCET READY (CH 042)":bool, "INTELLIFAUCET START (CH 043)":bool, "INTELLIFAUCET STOP (CH 044)":bool, "MAIN POWER RELAY (CH 047)":bool, "NOT USED (CH 045)":bool, "NOT USED (CH 046)":bool, "PURGE VALVE RELAY (CH 048)":bool, "OUTLET VALVE RELAY (CH 049)":bool, "INLET VALVE RELAY (CH 050)":bool, "Intellifaucet (% Open)":dbl, "Proportioning Valve (%Open)":dbl, "Intellifaucet Temp Setpoint (F)":dbl}
  T23 = typedef "Inficon Data.ctl" = cluster{"Gross Heating Value, Vol (Real, Dry)":dbl, "Nitrogen Component Normalized Mole % (Dry)":dbl, "Methane Component Normalized Mole % (Dry)":dbl, "Carbon Dioxide Component Normalized Mole % (Dry)":dbl, "Ethane Component Normalized Mole % (Dry)":dbl, "Propane Component Normalized Mole % (Dry)":dbl, "i-Pentane Component Normalized Mole % (Dry)":dbl, "i-Butane Component Normalized Mole % (Dry)":dbl, "n-Butane Component Normalized Mole % (Dry)":dbl, "n-Pentane Component Normalized Mole % (Dry)":dbl, "Hexane Component Normalized Mole % (Dry)":dbl, "Heptane Component Normalized Mole % (Dry)":dbl, "Gross Wobbe Index, Real(Dry)":dbl, "Relative Density, Real(Dry)":dbl, "Propylene Component Normalized Mole % (Dry)":dbl, "C4 Olefins Component Normalized Mole % (Dry)":dbl, "Water Component Normalized Mole % (Dry)":dbl}
  T24 = typedef "UTILITY Notifier.ctl" = enum16{"Set", "Read", "Release Ref"}
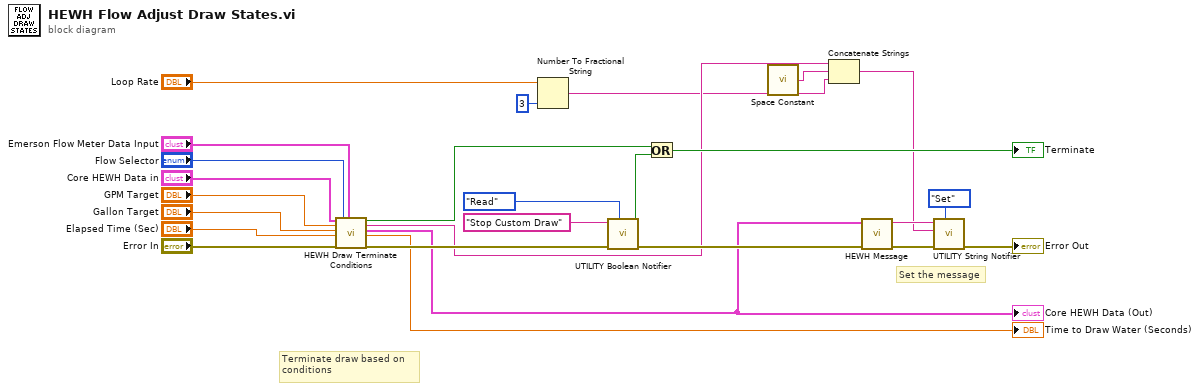
[diagram p0: block diagram]
diagram:
  # "Set the message"
  # "Terminate draw based on \nconditions"
  n1 = call "HEWH Draw Terminate Conditions.vi"("FileInit Cluster"="Core HEWH Data in", "GPM Target"="GPM Target", "Gallon Target"="Gallon Target", "Elapsed Time (Sec)"="Elapsed Time (Sec)", "Error In"="Error In", "Flow Selector"="Flow Selector", "Emerson Flow Meter Data Input"="Emerson Flow Meter Data Input") -> ("Terminate"=w26:bool, "Message"=w6:string, "FileInit Cluster Out"=w11:T4, "Time to Draw Water (Seconds)"=→"Time to Draw Water (Seconds)":T3, "Error Out"=w21:errorcluster)  [unwired: 8 in]
  "Core HEWH Data (Out)" <- w11
  n2 = Number To Fractional String(number="Loop Rate", precision (6)=i16 3) -> (F-format string=w4:string)  [unwired: 2 in]
  n3 = call "UTILITY Boolean Notifier.vi"("Status"=UTILITY_Notifier."Read", "error in (no error)"=w21, "name (unnamed)"="Stop Custom Draw") -> ("error out"=w13:errorcluster, "latest READ notification"=w23:bool)  [unwired: 7 in]
  n4 = Or(x=w26, y=w23) -> (x .or. y?=→"Terminate":bool)
  n5 = call <vilib>:"Space Constant.vi"() -> ("String"=w5:string)
  n6 = Concatenate Strings(w6, w5, w4) -> (w3:string)
  n7 = call "HEWH Message.vi"("Error In"=w13, "Core HEWH Data in"=w11) -> ("Error Out"=w12:errorcluster, "Message"=w14:string)  [unwired: 8 in]
  n8 = call "UTILITY String Notifier.vi"("Status"=UTILITY_Notifier."Set", "error in (no error)"=w12, "Set Status"=w3, "name (unnamed)"=w14) -> ("error out"=→"Error Out":errorcluster)  [unwired: 6 in, 1 out]
